vi "Periodic Tasks.vi"   [LabVIEW 2014]
doc: "This VI runs in parallel to other tasks. It can contain as many user-defined periodic loops as you need. These can carry out PID or other sorts of timed response."
uses:
  Robot Global Data.vi
  <vilib>/Rock Robotics/Network Tables/SD Write Number.vi
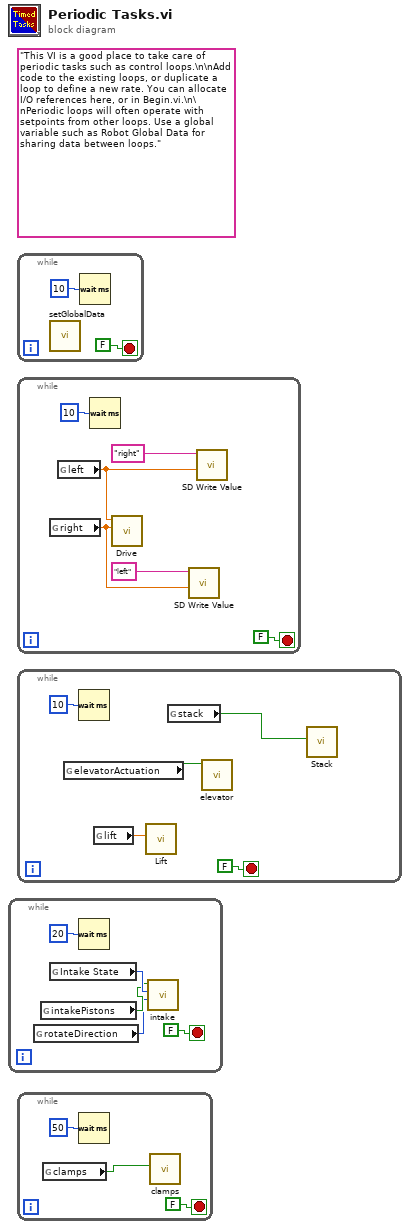
[diagram p0: block diagram]
diagram:
  (unwired) "This VI is a good place to take care of periodic tasks such as control loops.\n\nAdd code to the existing loops, or duplicate a loop to define a new rate. You can allocate I/O references here, or in Begin.vi.\n\nPeriodic loops will often operate with setpoints from other loops. Use a global variable such as Robot Global Data for sharing data between loops."
  n1 = while {
    stop <- FALSE stop-if-true
    n2 = global read "Robot Global Data.vi" "rotateDirection"() -> (w1:enum16{"left", "right"})
    n3 = global read "Robot Global Data.vi" "intakePistons"() -> (w2:bool)
    n4 = global read "Robot Global Data.vi" "Intake State"() -> (w3:enum16{"neutral", "rotate", "intake", "eject"})
    n5 = Wait (ms)(milliseconds to wait=u32 20) -> ()  [unwired: 1 out]
    n6 = call "intake.vi"("rotateDirection"=w1, "Intake State"=w3, "Intake"=w2) -> ()  [unwired: 9 in]
  }
  n7 = while {
    stop <- FALSE stop-if-true
    n8 = call "setGlobalData.vi"() -> ()  [unwired: 12 in]
    n9 = Wait (ms)(milliseconds to wait=u32 10) -> ()  [unwired: 1 out]
  }
  n10 = while {
    stop <- FALSE stop-if-true
    n11 = global read "Robot Global Data.vi" "right"() -> (w11:dbl)
    n12 = global read "Robot Global Data.vi" "left"() -> (w10:dbl)
    n13 = Wait (ms)(milliseconds to wait=u32 10) -> ()  [unwired: 1 out]
    n14 = call "Drive.vi"("right"=w11, "left"=w10) -> ()  [unwired: 10 in]
    n15 = call-poly <vilib>:"SD Write Value.vi"("Numeric"=w11, "Name"="left") -> ()  [unwired: 8 in, 2 out]
    n16 = call-poly <vilib>:"SD Write Value.vi"("Numeric"=w10, "Name"="right") -> ()  [unwired: 8 in, 2 out]
  }
  n17 = while {
    stop <- FALSE stop-if-true
    n18 = global read "Robot Global Data.vi" "elevatorActuation"() -> (w15:bool)
    n19 = Wait (ms)(milliseconds to wait=u32 10) -> ()  [unwired: 1 out]
    n20 = global read "Robot Global Data.vi" "lift"() -> (w16:dbl)
    n21 = call "Lift.vi"("lift"=w16) -> ()  [unwired: 11 in]
    n22 = global read "Robot Global Data.vi" "stack"() -> (w14:bool)
    n23 = call "elevator.vi"("Actuate?"=w15) -> ()  [unwired: 11 in]
    n24 = call "Stack.vi"("stack?"=w14) -> ()  [unwired: 11 in]
  }
  n25 = while {
    stop <- FALSE stop-if-true
    n26 = global read "Robot Global Data.vi" "clamps"() -> (w19:bool)
    n27 = Wait (ms)(milliseconds to wait=u32 50) -> ()  [unwired: 1 out]
    n28 = call "clamps.vi"("clamps"=w19) -> ()  [unwired: 11 in]
  }
